vi "Day02-1.vi"() -> ()   [LabVIEW 2021]
panel:
  out "x*y":i32
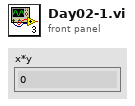
[diagram p1: front panel]
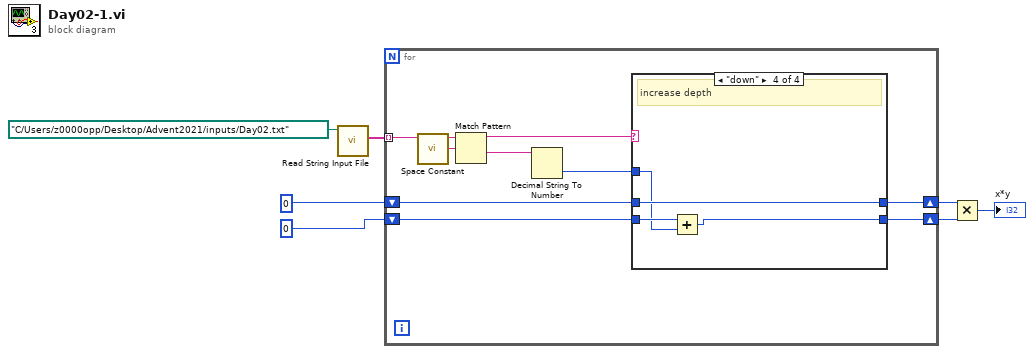
[diagram p0: block diagram]
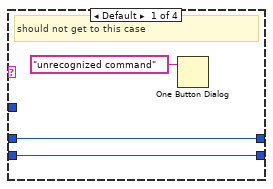
[diagram p2: hidden frame]
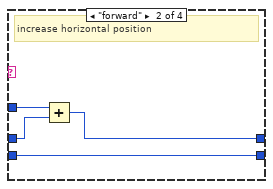
[diagram p3: hidden frame]
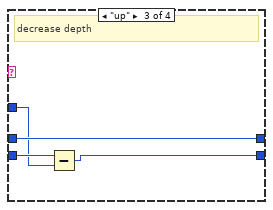
[diagram p4: hidden frame]
diagram:
  n1 = call "Read String Input File.vi"("file path (dialog if empty)"=path "C:/Users/z0000opp/Desktop/Advent2021/inputs/Day02.txt") -> ("input values"=w6:string[])  [unwired: 10 in]
  n2 = for {
    tunnel: w6 -> [w16] mode=indexing
    shift-right: [w8] -> w2
    shift-left: 0 -> [w12]
    shift-right: [w9] -> w3
    shift-left: 0 -> [w11]
    n3 = call <vilib>:"Space Constant.vi"() -> ("String"=w15:string)
    n4 = Match Pattern(string=w16, regular expression=w15) -> (before substring=w13:string, after substring=w14:string)  [unwired: 1 in, 2 out]
    n5 = Decimal String To Number(string=w14) -> (number=w10:i32)  [unwired: 2 in, 1 out]
    n6 = case shown="\"down\"" w13 {
      tunnel: w12 -> [w19 w20 w27 w31]
      tunnel: w11 -> [w18 w23 w26 w30]
      tunnel: w10 -> [_ w22 w24 w28]
      tunnel: [w18 w23 w25 w29] -> w9
      tunnel: [w19 w21 w27 w31] -> w8
      frame Default {
        # "should not get to this case"
        n7 = One Button Dialog(message="unrecognized command") -> ()  [unwired: 1 in, 1 out]
      }
      frame "forward" {
        # "increase horizontal position"
        n8 = Add(x=w22, y=w20) -> (x+y=w21:i32)
      }
      frame "up" {
        # "decrease depth"
        n9 = Subtract(x=w26, y=w24) -> (x-y=w25:i32)
      }
      frame "down" {
        # "increase depth"
        n10 = Add(x=w30, y=w28) -> (x+y=w29:i32)
      }
    }
  }
  n11 = Multiply(x=w2, y=w3) -> (x*y=→"x*y":i32)
